vi "LinxUartSetBaudRate.vi"(8 "Error In":errorcluster, 9 "Baud Rate":u32, 10 "Uart Channel":u8, 11 "LINX Resource":T1) -> (0 "Error Out":errorcluster, 1 "Actual Baud Rate":u32, 3 "LINX Resource":T1)   [LabVIEW 2020, in "LMH-LINX.lvlib" / "Local IO.lvlib"]
uses:
  Local IO.lvlib
  Type Defs/LINX Ref.ctl
  Type Defs/Platform.ctl
  Device/Type Defs/LINX Device Config.ctl
  Type Defs/Interface.ctl
  Device/Type Defs/TCP Config.ctl
  Device/Type Defs/Channels.ctl
  Type Defs/Error Type.ctl
  LMH-LINX.lvlib
  <vilib>/Instr/_visa.llb/VISA Configure Serial Port (Instr).vi
  myRIO/myRIO.lvlib
  Type Defs/Channel FGV States.ctl
  E:/lv2019/dist/vi.lib/MakerHub/LINX/Resources/liblinxdevice.dll
  Device/Device.lvlib
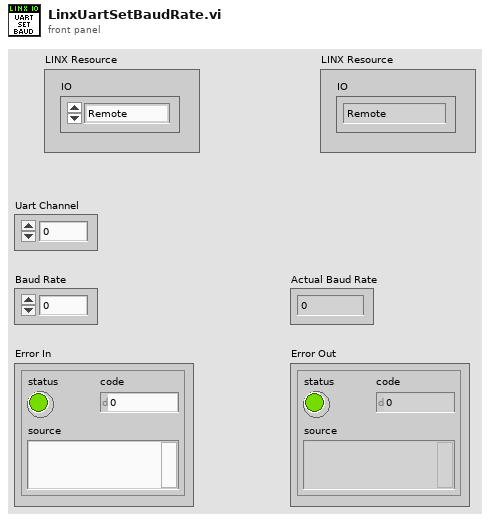
[diagram p1: front panel]
types:
  T1 = typedef "LMH-LINX.lvlib/LINX Ref.ctl" = cluster{"IO":T2, "LINX Device Config":T3}
  T2 = typedef "LMH-LINX.lvlib/Platform.ctl" = enum16{"Remote", "Local"}
  T3 = typedef "Device.lvlib/LINX Device Config.ctl" = cluster{"Interface":T4, "COM Port":refnum<visa-resource-name>, "TCP Configuration":T5, "Device Family":u8, "Device ID":u8, "Device Name":string, "TCP Ref":refnum<k5>, "Local Refnum":u64, "Channels":T6}
  T4 = typedef "LMH-LINX.lvlib/Interface.ctl" = enum16{"Serial", "TCP"}
  T5 = typedef "Device.lvlib/TCP Config.ctl" = cluster{"IP Address":string, "Port":u16}
  T6 = typedef "LMH-LINX.lvlib/Channels.ctl" = cluster{"DI":u8[], "DO":u8[], "AI":u8[], "AO":u8[], "PWM":u8[], "QE":u8[], "UART":u8[], "I2C 2":u8[], "SPI":u8[], "CAN":u8[], "Servo":u8[], "AI Ref (V)":dbl, "AI Resolution (Bits)":u8, "AO Ref (V)":dbl, "AO Resolution (Bits)":u8}
  T7 = typedef "LMH-LINX.lvlib/Error Type.ctl" = enum16{"Unknown", "Timeout", "Corrupt Return Packet", "Unable To Connect", "Command Not Supported", "Channel DNE", "Invalid COM Config", "Firmware Version Mismatch", "myRIO Support", "CMD Specific Error", "Local IO Not Supported"}
  T8 = typedef "LMH-LINX.lvlib/Channel FGV States.ctl" = enum16{"Initialize", "Get", "Set"}
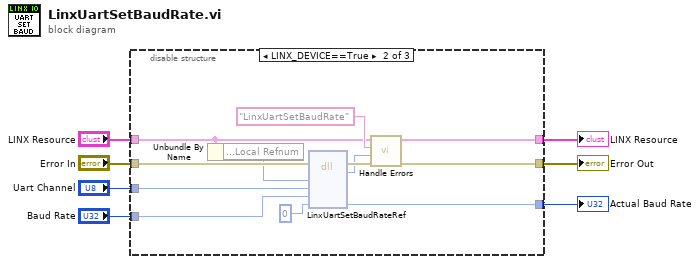
[diagram p0: block diagram]
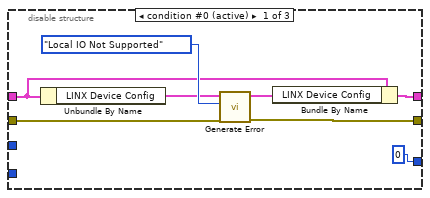
[diagram p2: hidden frame]
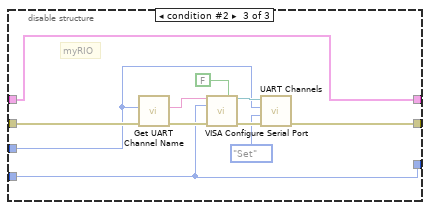
[diagram p3: hidden frame]
diagram:
  n1 = disable-structure shown="LINX_DEVICE==True" {
    disable-tunnel: [w9 w22 w31] -> w6
    disable-tunnel: "LINX Resource" -> [w11 w17 w31]
    disable-tunnel: "Error In" -> [w14 w27 w30]
    disable-tunnel: [w13 w20 w32] -> w7
    disable-tunnel: [u32 0 ("Baud Rate") w26 w29] -> w5
    disable-tunnel: "Uart Channel" -> [_ w24 w28]
    disable-tunnel: "Baud Rate" -> [_ w23 w29]
    frame condition #0 (active) {
      n2 = Unbundle By Name(w11) -> ("LINX Device Config"=w12:T3)
      n3 = call "Generate Error.vi"("Error In"=w14, "Error Type"=Error_Type."Local IO Not Supported", "LINX Device Config"=w12) -> ("Error Out"=w13:errorcluster, "Dup LINX Device Config"=w10:T3)  [unwired: 7 in]
      n4 = Bundle By Name(cluster=w11, "LINX Device Config"=w10) -> (w9:T1)
    }
    frame condition #1 {
      n5 = Unbundle By Name(w17) -> ("LINX Device Config.Local Refnum"=w16:u64)
      n6 = dll-call lib="E:/lv2019/dist/vi.lib/MakerHub/LINX/Resources/liblinxdevice.*" fn="LinxUartSetBaudRateRef"(error in=w27, "refnum"=w16, "channel"=w24, "baudRate"=w23, "actualBaud"=u32 0) -> (error out=w21:errorcluster, "status"=w18:i32, "actualBaud"=w26:u32)  [unwired: 5 in, 1 out]
      n7 = call "Handle Errors.vi"("Error In"=w21, "LinxStatus"=w18, "Function Name"="LinxUartSetBaudRate", "LINX Resource"=w17) -> ("Error Out"=w20:errorcluster, "LINX Resource"=w22:T1)  [unwired: 6 in]
    }
    frame condition #2 {
      # "myRIO"
      n8 = call "Get UART Channel Name.vi"("Error In"=w30, "UART Channel"=w28) -> ("Error Out"=w34:errorcluster, "UART Channel"=w35:string)  [unwired: 8 in]
      n9 = call-poly "VISA Configure Serial Port"("VISA resource name"=w35, "Enable Termination\nChar (T)"=FALSE ("Enable Termination\nChar (T)"), "baud rate (9600)"=w29, "error in (no error)"=w34) -> ("VISA resource name out"=w38:refnum<visa-resource-name>, "error out"=w37:errorcluster)  [unwired: 10 in]
      n10 = call "UART Channels.vi"("Error In"=w37, "Channel State"=Channel_FGV_States."Set", "Channel Number"=w28, "UART Channel"=w38) -> ("Error Out"=w32:errorcluster)  [unwired: 6 in, 1 out]
    }
  }
  "LINX Resource" <- w6
  "Actual Baud Rate" <- w5
  "Error Out" <- w7
